vi "InitFrontPanel.vi"(8 "ErrorArray In":errorcluster[](array[cluster])) -> (0 "ErrorArray Out":errorcluster[](array[cluster]))   [LabVIEW 2017, in "Framework.lvlib"]
uses:
  Framework.lvlib
  <vilib>/Utility/config.llb/Config Data RefNum.ctl
  Config_class/Config.lvclass/Config.ctl
  TypeDefs/clInitParams.ctl
  FrontPanel/TypeDefs/clEventConfig.ctl
  <vilib>/Utility/miscctls.llb/LVStringsAndValuesArrayTypeDef_U8.ctl
  Config_class/Accessors/Read ConfigFilePath.vi
  <vilib>/Utility/error.llb/Error Cluster From Error Code.vi
  <vilib>/ErrorRing/Error Ring.xnode
  <userlib>/NIST/NISTErrorLib/NISTErrorLib.lvlib
  Config_class/Config.lvclass
  <vilib>/Utility/config.llb/NI_LVConfig.lvlib
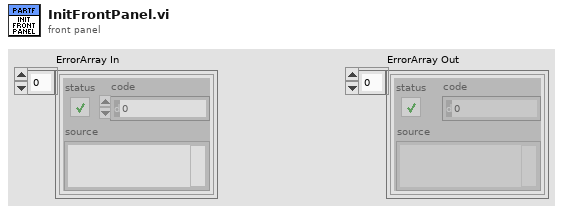
[diagram p1: front panel]
types:
  T1 = typedef "Framework.lvlib/clEventConfig.ctl" = cluster{"UTC Time 0":timestamp, "Nominal Frequency":u16, "Reporting Rate":u16, "Fsamp":u32, "PosSeq":bool}
  T2 = typedef "LVStringsAndValuesArrayTypeDef_U8.ctl" = cluster{"String":string, "Value":u8}[]
  T3 = typedef "NI_LVConfig.lvlib/Config Data RefNum.ctl" = refnum<k1>
  T4 = typedef "Framework.lvlib/clFrontPanelControlRefs.ctl" = cluster{"TestFilePathRef":refnum<vi>, "BusNumberRef":refnum<vi>, "NumberOfBusesRef":refnum<vi>, "EvtTypeRef":refnum<vi>, "EvtParamsRef":refnum<vi>, "EvtConfigRef":refnum<vi>, "StartTimeRef":refnum<vi>, "EndTimeRef":refnum<vi>, "PmuImpairTypeRef":refnum<vi>, "PmuImpairParamsRef":refnum<vi>, "NetImpairParamsRef":refnum<vi>, "FlagImpairTypeRef":refnum<vi>, "FlagImpairParamsRef":refnum<vi>, "NetImpairTypeRef":refnum<vi>, "OutputFileType":refnum<vi>, "PmuImpairConfigRef":refnum<vi>, "AppTypeRef":refnum<vi>, "ScriptPathRef":refnum<vi>, "ShowPanels?":refnum<vi>}
  T5 = typedef "Framework.lvlib/clInitParams.ctl" = cluster{"RowHdrs":string[], "ColHdrs":string[], "DefaultParams":string[][]}
  T6 = typedef "PmuImpairPlugins.lvlib/PmuImpairPluginBase.lvclass/clImpairConfig.ctl" = cluster{"FilterType":string, "bPosSeq":bool}
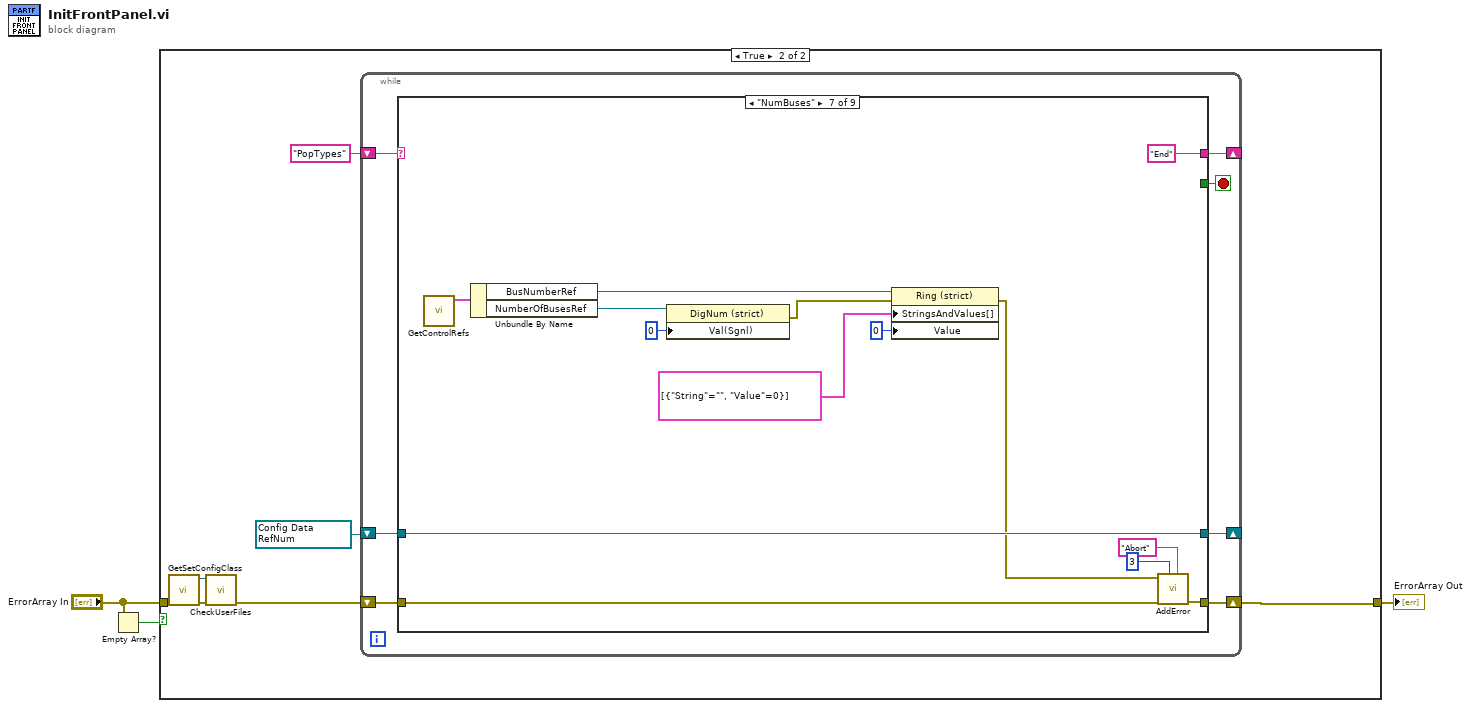
[diagram p0: block diagram]
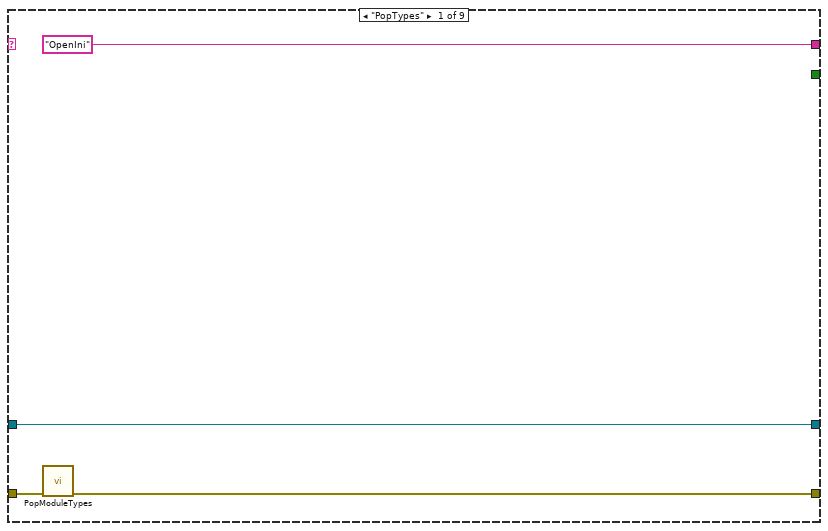
[diagram p3: hidden frame]
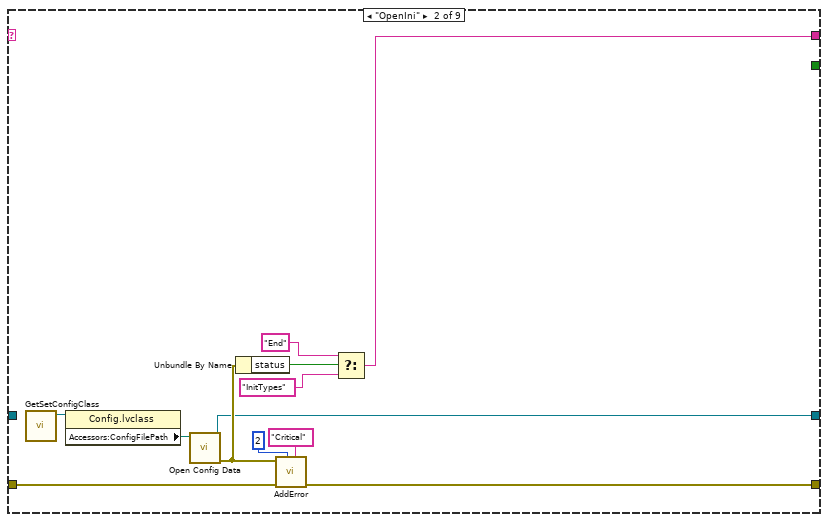
[diagram p4: hidden frame]
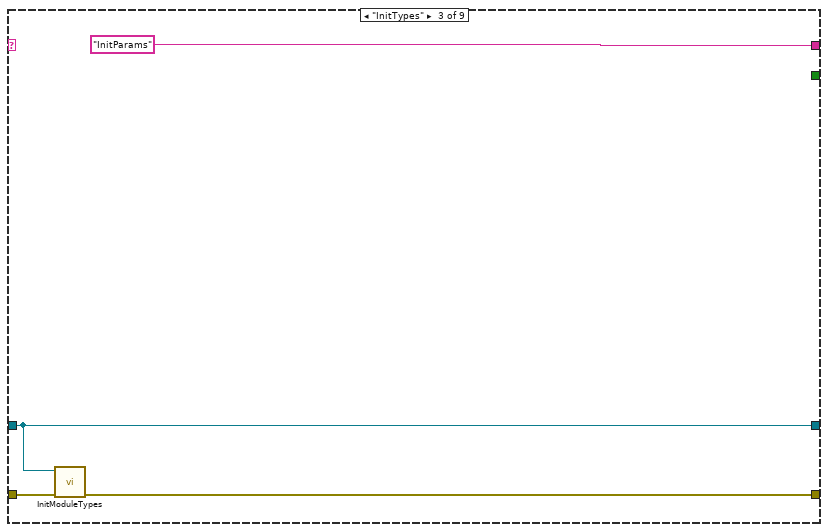
[diagram p5: hidden frame]
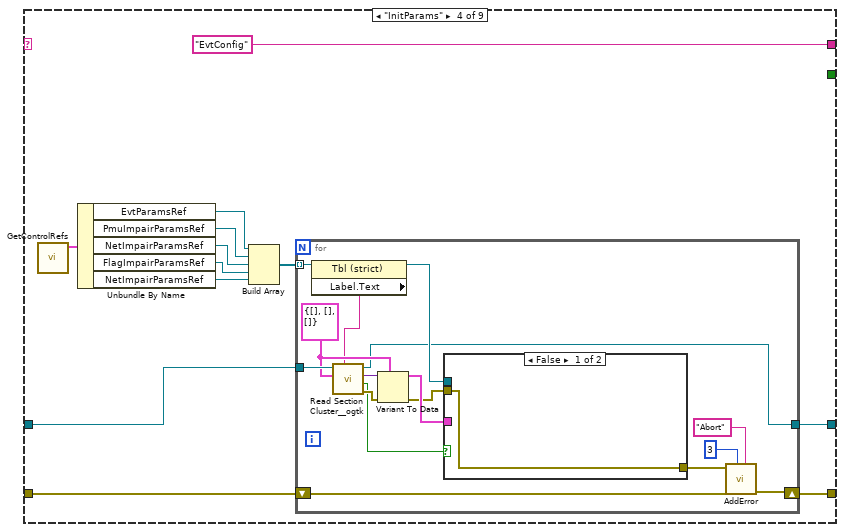
[diagram p6: hidden frame]
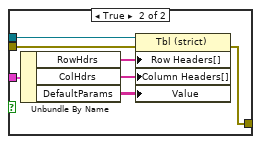
[diagram p7: hidden frame]
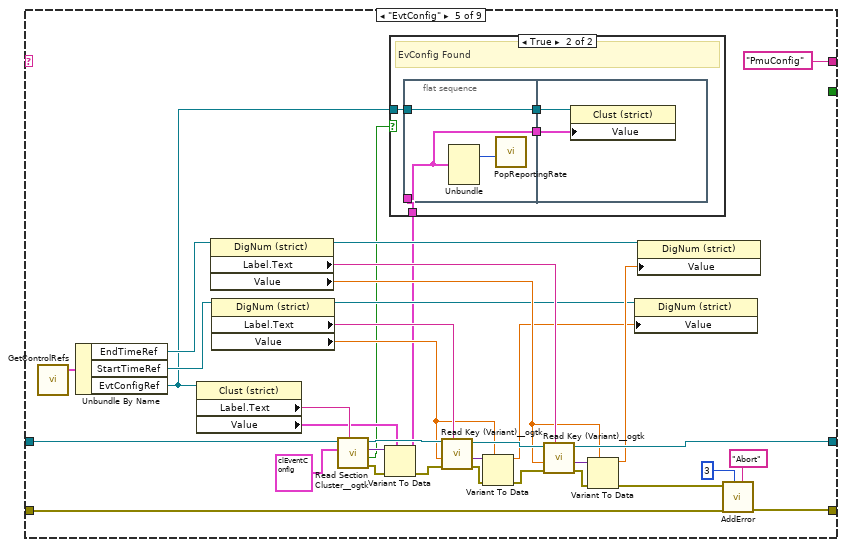
[diagram p8: hidden frame]
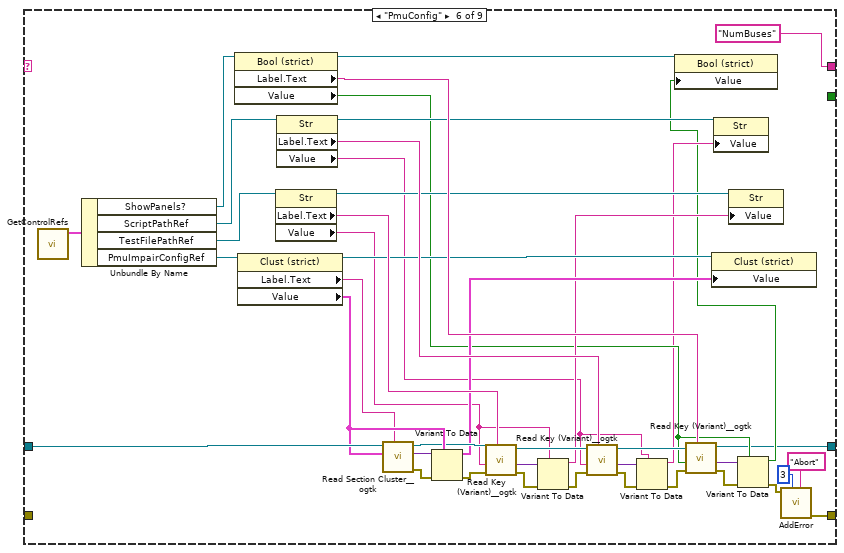
[diagram p10: hidden frame]
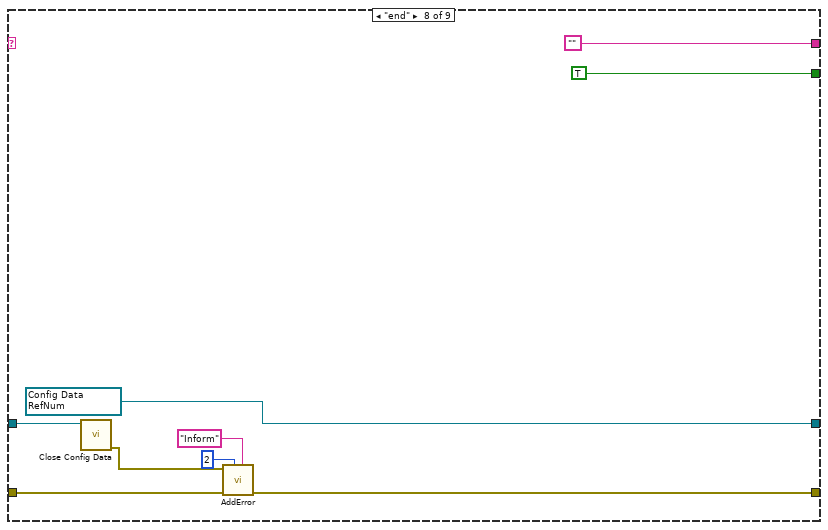
[diagram p11: hidden frame]
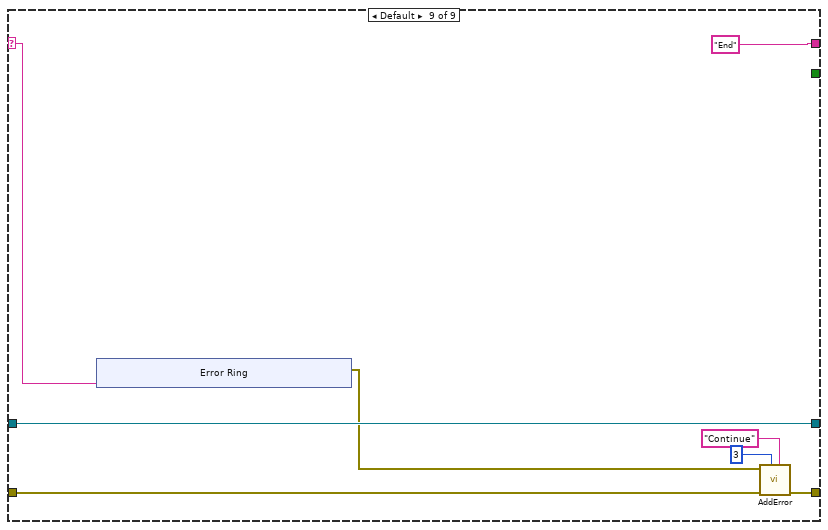
[diagram p12: hidden frame]
diagram:
  n1 = Empty Array?(array="ErrorArray In") -> (empty?=w2:bool)
  n2 = case shown="True" w2 {
    tunnel: "ErrorArray In" -> [w5 w11]
    tunnel: [w4 w8] -> w3
    frame False {
      n3 = call <userlib>:"AddError.vi"("ErrorArray"=w5) -> ("ErrorArray"=w4:errorcluster[])  [unwired: 9 in, 1 out]
    }
    frame True {
      w6 = T3 refnum items=["config data"] ("refnum")
      n4 = call "GetSetConfigClass.vi"() -> ("Ref out"=w10:refnum<class "Config.lvclass">)  [unwired: 11 in]
      n5 = call "CheckUserFiles.vi"("ErrorArray"=w11, "Config in"=w10) -> ("ErrorArray"=w9:errorcluster[])  [unwired: 8 in, 1 out]
      n6 = while {
        shift-right: [w16] -> _
        shift-left: "PopTypes" -> [w18]
        shift-right: [w14] -> w8
        shift-left: w9 -> [w17]
        shift-right: [w13] -> _
        shift-left: w6 -> [w12]
        stop <- w15 stop-if-true
        n7 = case shown="\"NumBuses\"" w18 {
          selector: w18 -> [_ _ _ _ _ _ _ _ w191]
          tunnel: w17 -> [w22 w32 w37 w41 w79 _ w161 w181 w187]
          tunnel: ["OpenIni" w24 "InitParams" "EvtConfig" "PmuConfig" "NumBuses" "End" "" "End"] -> w16
          tunnel: [_ _ _ _ _ _ _ TRUE _] -> w15
          tunnel: [w20 w29 w36 w40 w78 w122 w166 w178 w190] -> w14
          tunnel: [w19 w23 w35 w42 w93 w123 w165 w179 w189] -> w13
          tunnel: w12 -> [w19 _ w35 w43 w105 w154 w165 w180 w189]
          frame "PopTypes" {
            n8 = call "PopModuleTypes.vi"("ErrorArray In"=w22) -> ("ErrorArray Out"=w20:errorcluster[])  [unwired: 10 in]
          }
          frame "OpenIni" {
            n9 = call "GetSetConfigClass.vi"() -> ("Ref out"=w34:refnum<class "Config.lvclass">)  [unwired: 11 in]
            n10 = property class="Config.lvclass"(reference=w34) -> ("Accessors:ConfigFilePath"=w33:path)  [unwired: 1 in, 2 out]
            n11 = call <vilib>:"Open Config Data.vi"("configuration file path"=w33) -> ("error out"=w28:errorcluster, "refnum"=w23:T3)  [unwired: 8 in, 1 out]
            n12 = Unbundle By Name(w28) -> ("status"=w27:bool)
            n13 = call <userlib>:"AddError.vi"("Severity"="Critical", "Priority"=u8 2, "ErrorArray"=w32, "error in (no error)"=w28) -> ("ErrorArray"=w29:errorcluster[])  [unwired: 6 in, 1 out]
            n14 = Select(t="End", s=w27, f="InitTypes") -> (s? t:f=w24:string)
          }
          frame "InitTypes" {
            n15 = call "InitModuleTypes.vi"("ErrorArray In"=w37, "refnum"=w35) -> ("ErrorArray Out"=w36:errorcluster[])  [unwired: 9 in]
          }
          frame "InitParams" {
            n16 = call "GetControlRefs.vi"() -> ("clControlRefs Out"=w50:T4)  [unwired: 11 in]
            n17 = Unbundle By Name(w50) -> ("EvtParamsRef"=w45:refnum<vi>, "PmuImpairParamsRef"=w46:refnum<vi>, "NetImpairParamsRef"=w47:refnum<vi>, "FlagImpairParamsRef"=w48:refnum<vi>, "NetImpairParamsRef"=w49:refnum<vi>)
            n18 = Build Array(w45, w46, w47, w48, w49) -> (w44:refnum<vi>[])
            n19 = for {
              tunnel: w44 -> [w61] mode=indexing
              tunnel: w43 -> [w64]
              tunnel: [w57] -> w42
              shift-right: [w55] -> w40
              shift-left: w41 -> [w56]
              w63 = T5 {"RowHdrs"=[], "ColHdrs"=[], "DefaultParams"=[]} ("ParamsHdrs")
              n20 = property class="Tbl (strict)"(reference=w61) -> (reference out=w59:refnum<vi>, "Label.Text"=w60:string)  [unwired: 1 in, 1 out]
              n21 = call <userlib>:"Read Section Cluster__ogtk.vi"("section (optional)"=w60, "Section Formatted Cluster Type"=w63, "refnum"=w64) -> ("error out"=w66:errorcluster, "all found?"=w51:bool, "Section Formatted Cluster"=w65:variant, "dup refnum"=w57:T3)  [unwired: 4 in, 1 out]
              n22 = Variant To Data(error in=w66, type=w63, Variant=w65) -> (data=w62:T5, error out=w58:errorcluster)
              n23 = case shown="False" w51 {
                tunnel: w62 -> [_ w74]
                tunnel: w59 -> [_ w72]
                tunnel: w58 -> [w67 w71]
                tunnel: [w67 w70] -> w54
                frame False {
                }
                frame True {
                  n24 = Unbundle By Name(w74) -> ("RowHdrs"=w68:string[], "ColHdrs"=w69:string[], "DefaultParams"=w73:string[][])
                  n25 = property on="Property Node" class="Tbl (strict)"(reference=w72, error in=w71, "Row Headers[]"=w68, "Column Headers[]"=w69, "Value"=w73) -> (error out=w70:errorcluster)  [unwired: 1 out]
                }
              }
              n26 = call <userlib>:"AddError.vi"("Severity"="Abort", "Priority"=u8 3, "ErrorArray"=w56, "error in (no error)"=w54) -> ("ErrorArray"=w55:errorcluster[])  [unwired: 6 in, 1 out]
            }
          }
          frame "EvtConfig" {
            n27 = call "GetControlRefs.vi"() -> ("clControlRefs Out"=w108:T4)  [unwired: 11 in]
            n28 = Unbundle By Name(w108) -> ("EndTimeRef"=w106:refnum<vi>, "StartTimeRef"=w107:refnum<vi>, "EvtConfigRef"=w81:refnum<vi>)
            n29 = property class="Clust (strict)"(reference=w81) -> ("Label.Text"=w104:string, "Value"=w84:T1)  [unwired: 1 in, 2 out]
            n30 = property class="DigNum (strict)"(reference=w106) -> (reference out=w92:refnum<vi>, "Label.Text"=w102:string, "Value"=w91:dbl)  [unwired: 1 in, 1 out]
            n31 = property class="DigNum (strict)"(reference=w107) -> (reference out=w88:refnum<vi>, "Label.Text"=w103:string, "Value"=w89:dbl)  [unwired: 1 in, 1 out]
            n32 = call <userlib>:"Read Section Cluster__ogtk.vi"("section (optional)"=w104, "Section Formatted Cluster Type"=T1 {"UTC Time 0"=timestamp(0 s since 1904-01-01), "Nominal Frequency"=60, "Reporting Rate"=60, "Fsamp"=960, "PosSeq"=FALSE} ("Value"), "refnum"=w105) -> ("error out"=w101:errorcluster, "all found?"=w83:bool, "Section Formatted Cluster"=w100:variant, "dup refnum"=w99:T3)  [unwired: 4 in, 1 out]
            n33 = Variant To Data(error in=w101, type=w84, Variant=w100) -> (data=w82:T1, error out=w86:errorcluster)
            n34 = case shown="True" w83 {
              tunnel: w82 -> [_ w113]
              tunnel: w81 -> [_ w112]
              frame False {
                # "EvtConfig Not Found"
              }
              frame True {
                # "EvConfig Found"
                n35 = flat-sequence {
                  tunnel: w113 -> [w114]
                  tunnel: w112 -> [w115]
                  tunnel: [w115] -> w111
                  tunnel: [w114] -> w110
                  tunnel: w111 -> [w118]
                  tunnel: w110 -> [w117]
                  frame #0 {
                    n36 = Unbundle(w114) -> ("Nominal Frequency"=w116:u16)  [unwired: 4 out]
                    n37 = call "PopReportingRate.vi"("Nominal Frequency (60)"=w116) -> ()  [unwired: 10 in, 1 out]
                  }
                  frame #1 {
                    n38 = property class="Clust (strict)"(reference=w118, "Value"=w117) -> ()  [unwired: 1 in, 2 out]
                  }
                }
              }
            }
            n39 = call <userlib>:"Read Key (Variant)__ogtk.vi"("section"=w103, "error in (no error)"=w86, "type"=w89, "refnum"=w99) -> ("error out"=w98:errorcluster, "key-value"=w97:variant, "refnum out"=w94:T3)  [unwired: 4 in, 1 out]
            n40 = Variant To Data(error in=w98, type=w89, Variant=w97) -> (data=w87:dbl, error out=w85:errorcluster)
            n41 = call <userlib>:"Read Key (Variant)__ogtk.vi"("section"=w102, "error in (no error)"=w85, "type"=w91, "refnum"=w94) -> ("error out"=w96:errorcluster, "key-value"=w95:variant, "refnum out"=w93:T3)  [unwired: 4 in, 1 out]
            n42 = Variant To Data(error in=w96, type=w91, Variant=w95) -> (data=w90:dbl, error out=w80:errorcluster)
            n43 = property class="DigNum (strict)"(reference=w88, "Value"=w87) -> ()  [unwired: 1 in, 2 out]
            n44 = property class="DigNum (strict)"(reference=w92, "Value"=w90) -> ()  [unwired: 1 in, 2 out]
            n45 = call <userlib>:"AddError.vi"("Severity"="Abort", "Priority"=u8 3, "ErrorArray"=w79, "error in (no error)"=w80) -> ("ErrorArray"=w78:errorcluster[])  [unwired: 6 in, 1 out]
          }
          frame "PmuConfig" {
            n46 = call "GetControlRefs.vi"() -> ("clControlRefs Out"=w159:T4)  [unwired: 11 in]
            n47 = Unbundle By Name(w159) -> ("ShowPanels?"=w158:refnum<vi>, "ScriptPathRef"=w157:refnum<vi>, "TestFilePathRef"=w156:refnum<vi>, "PmuImpairConfigRef"=w155:refnum<vi>)
            n48 = property class="Bool (strict)"(reference=w158) -> (reference out=w131:refnum<vi>, "Label.Text"=w135:string, "Value"=w126:bool)  [unwired: 1 in, 1 out]
            n49 = property class="Clust (strict)"(reference=w155) -> (reference out=w134:refnum<vi>, "Label.Text"=w138:string, "Value"=w151:T6)  [unwired: 1 in, 1 out]
            n50 = property class="Str"(reference=w156) -> (reference out=w133:refnum<vi>, "Label.Text"=w137:string, "Value"=w128:string)  [unwired: 1 in, 1 out]
            n51 = property class="Str"(reference=w157) -> (reference out=w132:refnum<vi>, "Label.Text"=w136:string, "Value"=w127:string)  [unwired: 1 in, 1 out]
            n52 = call <userlib>:"Read Section Cluster__ogtk.vi"("section (optional)"=w138, "Section Formatted Cluster Type"=w151, "refnum"=w154) -> ("error out"=w153:errorcluster, "Section Formatted Cluster"=w152:variant, "dup refnum"=w149:T3)  [unwired: 4 in, 2 out]
            n53 = Variant To Data(error in=w153, type=w151, Variant=w152) -> (data=w130:T6, error out=w150:errorcluster)
            n54 = call <userlib>:"Read Key (Variant)__ogtk.vi"("section"=w137, "error in (no error)"=w150, "type"=w128, "refnum"=w149) -> ("error out"=w148:errorcluster, "key-value"=w147:variant, "refnum out"=w140:T3)  [unwired: 4 in, 1 out]
            n55 = Variant To Data(error in=w148, type=w128, Variant=w147) -> (data=w129:string, error out=w144:errorcluster)
            n56 = call <userlib>:"Read Key (Variant)__ogtk.vi"("section"=w136, "error in (no error)"=w144, "type"=w127, "refnum"=w140) -> ("error out"=w145:errorcluster, "key-value"=w146:variant, "refnum out"=w139:T3)  [unwired: 4 in, 1 out]
            n57 = Variant To Data(error in=w145, type=w127, Variant=w146) -> (data=w125:string, error out=w141:errorcluster)
            n58 = call <userlib>:"Read Key (Variant)__ogtk.vi"("section"=w135, "error in (no error)"=w141, "type"=w126, "refnum"=w139) -> ("error out"=w143:errorcluster, "key-value"=w142:variant, "refnum out"=w123:T3)  [unwired: 4 in, 1 out]
            n59 = property class="Clust (strict)"(reference=w134, "Value"=w130) -> ()  [unwired: 1 in, 2 out]
            n60 = property class="Str"(reference=w132, "Value"=w125) -> ()  [unwired: 1 in, 2 out]
            n61 = property class="Str"(reference=w133, "Value"=w129) -> ()  [unwired: 1 in, 2 out]
            n62 = Variant To Data(error in=w143, type=w126, Variant=w142) -> (data=w124:bool, error out=w121:errorcluster)
            n63 = property class="Bool (strict)"(reference=w131, "Value"=w124) -> ()  [unwired: 1 in, 2 out]
            n64 = call <userlib>:"AddError.vi"("Severity"="Abort", "Priority"=u8 3, "error in (no error)"=w121) -> ("ErrorArray"=w122:errorcluster[])  [unwired: 7 in, 1 out]
          }
          frame "NumBuses" {
            n65 = call "GetControlRefs.vi"() -> ("clControlRefs Out"=w167:T4)  [unwired: 11 in]
            n66 = Unbundle By Name(w167) -> ("BusNumberRef"=w170:refnum<vi>, "NumberOfBusesRef"=w168:refnum<vi>)
            n67 = property class="DigNum (strict)"(reference=w168, "Val(Sgnl)"=u8 0 ("Value")) -> (error out=w171:errorcluster)  [unwired: 1 in, 1 out]
            n68 = property class="Ring (strict)"(reference=w170, error in=w171, "StringsAndValues[]"=T2 [{"String"="", "Value"=0}] ("Strings And Values []"), "Value"=u8 0) -> (error out=w164:errorcluster)  [unwired: 1 out]
            n69 = call <userlib>:"AddError.vi"("Severity"="Abort", "Priority"=u8 3, "ErrorArray"=w161, "error in (no error)"=w164) -> ("ErrorArray"=w166:errorcluster[])  [unwired: 6 in, 1 out]
          }
          frame "end" {
            w179 = T3 refnum items=["config data"] ("refnum")
            n70 = call <vilib>:"Close Config Data.vi"("refnum"=w180) -> ("error out"=w177:errorcluster)  [unwired: 9 in, 1 out]
            n71 = call <userlib>:"AddError.vi"("Severity"="Inform", "Priority"=u8 2, "ErrorArray"=w181, "error in (no error)"=w177) -> ("ErrorArray"=w178:errorcluster[])  [unwired: 6 in, 1 out]
          }
          frame Default {
            n72 = xnode "Error Ring"("parameter 0"=w191) -> ("error out"=w186:errorcluster)
            n73 = call <userlib>:"AddError.vi"("Severity"="Continue", "Priority"=u8 3, "ErrorArray"=w187, "error in (no error)"=w186) -> ("ErrorArray"=w190:errorcluster[])  [unwired: 6 in, 1 out]
          }
        }
      }
    }
  }
  "ErrorArray Out" <- w3
